vi "Spartan Server Shutdown.vi"(4 "error in (no error)":errorcluster) -> (0 "error out":errorcluster)   [LabVIEW 2011]
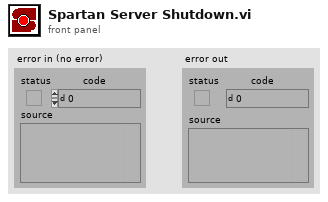
[diagram p1: front panel]
types:
  T1 = typedef "Connection Refnum.ctl" = cluster{"Environment Handle":i32, "Connection Handle":i32}
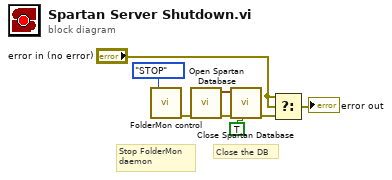
[diagram p0: block diagram]
diagram:
  # "Close the DB"
  # "Stop FolderMon\ndaemon"
  n1 = call "FolderMon control.vi"("Action (START)"=enum16{"START", "STOP"}."STOP") -> ("error out"=w4:errorcluster)  [unwired: 2 in, 4 out]
  n2 = call "Open Spartan Database.vi"("error in (no error)"=w4) -> ("error out"=w3:errorcluster, "Connection Refnum"=w2:T1)  [unwired: 1 in, 8 out]
  n3 = call "Close Spartan Database.vi"("Force Close? (f)"=TRUE ("Server Close? (f)"), "error in (no error)"=w3, "Connection Refnum"=w2) -> ("error out"=w1:errorcluster)  [unwired: 2 in, 6 out]
  n4 = Select(t="error in (no error)", s="error in (no error)", f=w1) -> (s? t:f=→"error out":errorcluster)
